vi "Scalar_Data.vi"() -> ()   [LabVIEW 2012]
panel:
  out "Scalar Data":u16[](array[numeric])
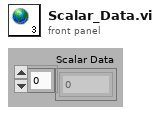
[diagram p1: front panel]
diagram:
